vi "SECS Request.vi"(8 "error in (no error)":errorcluster, 10 "Scenarios Class":refnum<class "Scenarios Class.lvclass">, 11 "Scenarios Class in":refnum<class "Scenarios Class.lvclass">) -> (0 "error out":errorcluster, 3 "Scenarios Class out":refnum<class "Scenarios Class.lvclass">)   [LabVIEW 2020, in "SECS Scenarios.lvlib" / "Scenarios Class.lvclass"]
uses:
  Scenarios Class.lvclass
  Scenarios Class.lvclass/Scenarios Class.ctl
  Write HSMS Class.vi
  Write On-Line Notifier.vi
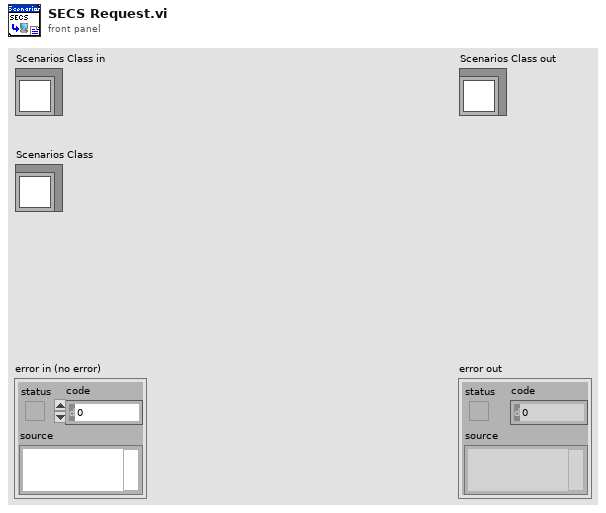
[diagram p1: front panel]
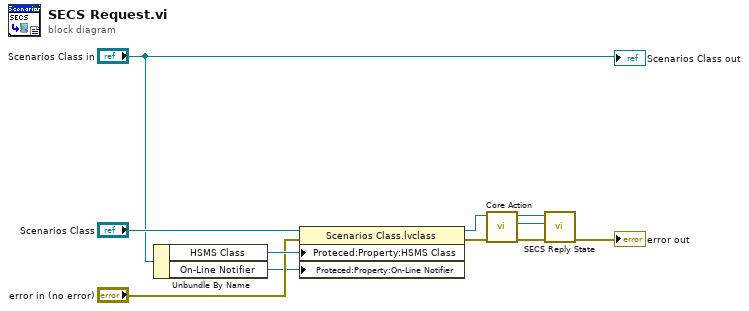
[diagram p0: block diagram]
diagram:
  n1 = Unbundle By Name("Scenarios Class in") -> ("HSMS Class"=w11:refnum<class "HSMS Class.lvclass">, "On-Line Notifier"=w1:refnum<notifier>)
  n2 = property class="Scenarios Class.lvclass"(reference="Scenarios Class", error in="error in (no error)", "Proteced:Property:HSMS Class"=w11, "Proteced:Property:On-Line Notifier"=w1) -> (reference out=w10:refnum<class "Scenarios Class.lvclass">, error out=w9:errorcluster)
  n3 = call-dynamic "Core Action.vi"("error in (no error)"=w9, "Scenarios Class in"=w10) -> ("error out"=w6:errorcluster, "SECS-II Class Out"=w2:refnum<class "SECS-II Class.lvclass">, "Scenarios Class out"=w4:refnum<class "Scenarios Class.lvclass">)  [unwired: 7 in]
  n4 = call "SECS Reply State.vi"("error in (no error)"=w6, "SECS-II Class In"=w2, "Scenarios Class in"=w4) -> ("error out"=→"error out":errorcluster)  [unwired: 7 in, 1 out]
  "Scenarios Class out" <- "Scenarios Class in"
